vi "Insert Initial Delay - IQ.vi"(0 "data in":T1[](array[typedef])=[{"I"=0.0, "Q"=0.0, "overflow"=FALSE}, {"I"=0.0, "Q"=0.0, "overflow"=FALSE}, {"I"=0.0, "Q"=0.0, "overflow"=FALSE}, {"I"=0.0, "Q"=0.0, "overflow"=FALSE}], 1 "insert":bool, 2 "reset":bool, 9 "input valid":bool, 11 "delay":u32) -> (3 "done":bool, 4 "data out":T1[](array[typedef]), 10 "output valid":bool)   [LabVIEW 2018, in "GettingStarted_5774_FPGA.lvlib"]
doc: "Inserts initial idle samples in the sample stream.\n\nA true on the <B>reset</B> input resets the internal state machine and sets the <B>output valid</B> and <B>done</B> outputs to false. Following a reset the VI waits until it detects a rising edge on the <B>insert</B> input which initiates the idle sample insertion. During this period <B>delay</B> number of idle samples are returned on the <B>data output</B>. When no more idle samples can be returned (because the remaining number of idle samples is less than the number of samples returned on the <B>data out</B> output) the <B>done</B> output is set to true and the VI starts returning the samples provided on the <B>data in</B> input. The <B>data in</B> input is ignored if the <B>done</B> output was false in the previous cycle.\n\nSupported array size of the <B>data in</B> input: 1, 2, 4, 8, 16 or 32.\nThe data pipeline delay of this VI is 1 clock cycle."
uses:
  <instrlib>/_niInstr/DSP/v1/Shared/Public/IQ Data.ctl
  <instrlib>/_niInstr/Basic Elements/v1/FPGA/Private/Count Down U32.vi
  GettingStarted_5774_FPGA.lvlib
  <instrlib>/_niInstr/DSP/v1/Shared/niInstr DSP v1 Shared.lvlib
  <instrlib>/_niInstr/Basic Elements/v1/FPGA/niInstr Basic Elements v1 FPGA.lvlib
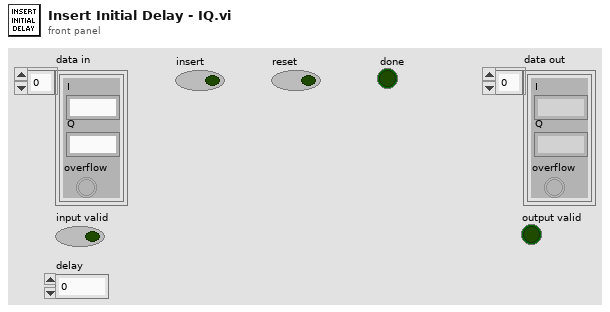
[diagram p1: front panel]
types:
  T1 = typedef "niInstr DSP v1 Shared.lvlib/IQ Data.ctl" = cluster{"I":fxp<+/-,18,1>, "Q":fxp<+/-,18,1>, "overflow":bool}
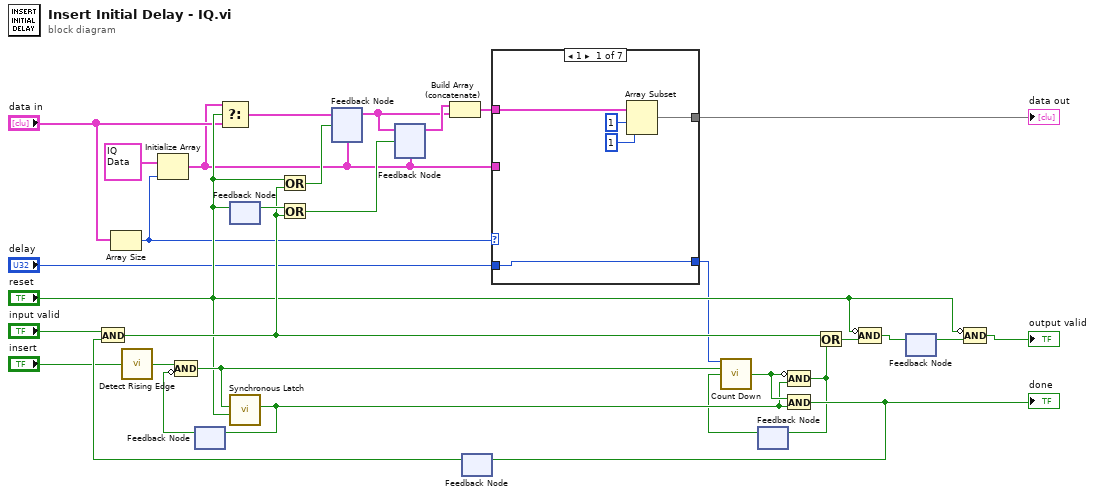
[diagram p0: block diagram]
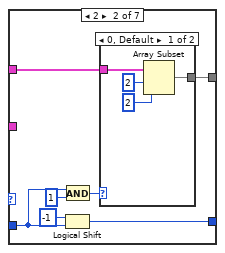
[diagram p2: hidden frame]
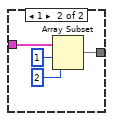
[diagram p3: hidden frame]
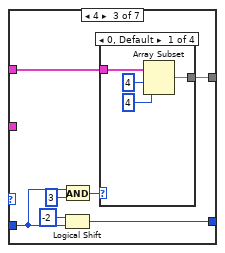
[diagram p4: hidden frame]
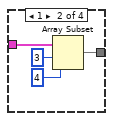
[diagram p5: hidden frame]
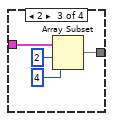
[diagram p6: hidden frame]
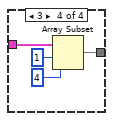
[diagram p7: hidden frame]
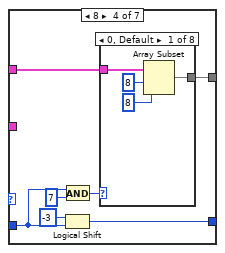
[diagram p8: hidden frame]
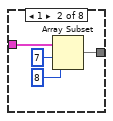
[diagram p9: hidden frame]
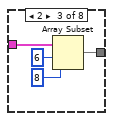
[diagram p10: hidden frame]
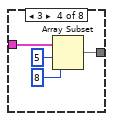
[diagram p11: hidden frame]
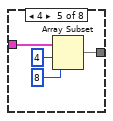
[diagram p12: hidden frame]
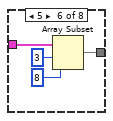
[diagram p13: hidden frame]
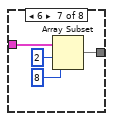
[diagram p14: hidden frame]
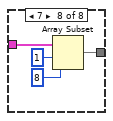
[diagram p15: hidden frame]
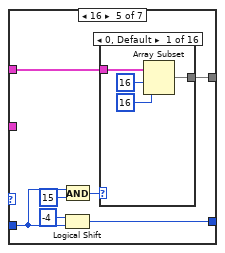
[diagram p16: hidden frame]
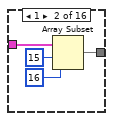
[diagram p17: hidden frame]
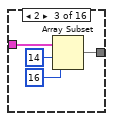
[diagram p18: hidden frame]
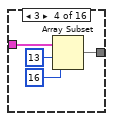
[diagram p19: hidden frame]
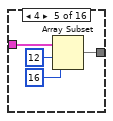
[diagram p20: hidden frame]
diagram:
  n1 = Array Size(array="data in") -> (size(s)=w6:i32)
  n2 = call <instrlib>:"Detect Rising Edge.vi"("signal"="insert") -> ("edge detected"=w19:bool)  [unwired: 14 in]
  n3 = Initialize Array(T1 {"I"=0.0, "Q"=0.0, "overflow"=FALSE} ("data"), w6) -> (w1:T1[])
  n4 = feedback #1() -> (w17:bool)  [unwired: 1 in]
  n5 = Compound Arithmetic op=AND(w19, invert w17) -> (w18:bool)
  n6 = Select(t=w1, s="reset", f="data in") -> (s? t:f=w30:T1[])
  n7 = feedback-in #2("reset") -> ()
  n8 = feedback #2() -> (w27:bool)  [unwired: 1 in]
  n9 = call <instrlib>:"Synchronous Latch.vi"("clear"="reset", "set"=w18) -> ("out"=w16:bool)  [unwired: 9 in]
  n10 = feedback-in #1(w16) -> ()
  n11 = feedback #3(w1) -> (w23:T1[])
  n12 = feedback #4(w1) -> (w24:T1[])
  n13 = Build Array (concatenate)(w24, w23) -> (w4:T1[])
  n14 = feedback #5() -> (w25:bool)  [unwired: 1 in]
  n15 = And(x="input valid", y=w25) -> (x .and. y?=w15:bool)
  n16 = Or(x="reset", y=w15) -> (x .or. y?=w28:bool)
  n17 = Or(x=w27, y=w15) -> (x .or. y?=w26:bool)
  n18 = feedback-in #3(w30, w28) -> ()
  n19 = feedback-in #4(w23, w26) -> ()
  n20 = case shown="1" w6 {
    tunnel: "delay" -> [w34 w42 w57 w80 w119 w190 w324]
    tunnel: w4 -> [w36 w39 w54 w77 w116 w187 _]
    tunnel: [w34 w38 w53 w76 w115 w186 w324] -> w3
    tunnel: [w35 w37 w52 w75 w114 w185 w323] -> w2
    tunnel: w1 -> [_ _ _ _ _ _ w323]
    frame 1 {
      n21 = Array Subset(array=w36, index=1, length=1) -> (w35:T1[])
    }
    frame 2 {
      n22 = Logical Shift(y=i16 -1, x=w42) -> (x << y=w38:u32)
      n23 = And(x=w42, y=u32 1) -> (x .and. y?=w40:u32)
      n24 = case shown="0, Default" w40 {
        tunnel: w39 -> [w47 w51]
        tunnel: [w46 w50] -> w37
        frame 0, Default {
          n25 = Array Subset(array=w47, index=2, length=2) -> (w46:T1[])
        }
        frame 1 {
          n26 = Array Subset(array=w51, index=1, length=2) -> (w50:T1[])
        }
      }
    }
    frame 4 {
      n27 = Logical Shift(y=i16 -2, x=w57) -> (x << y=w53:u32)
      n28 = And(x=w57, y=u32 3) -> (x .and. y?=w55:u32)
      n29 = case shown="0, Default" w55 {
        tunnel: w54 -> [w62 w66 w70 w74]
        tunnel: [w61 w65 w69 w73] -> w52
        frame 0, Default {
          n30 = Array Subset(array=w62, index=4, length=4) -> (w61:T1[])
        }
        frame 1 {
          n31 = Array Subset(array=w66, index=3, length=4) -> (w65:T1[])
        }
        frame 2 {
          n32 = Array Subset(array=w70, index=2, length=4) -> (w69:T1[])
        }
        frame 3 {
          n33 = Array Subset(array=w74, index=1, length=4) -> (w73:T1[])
        }
      }
    }
    frame 8 {
      n34 = Logical Shift(y=i16 -3, x=w80) -> (x << y=w76:u32)
      n35 = And(x=w80, y=u32 7) -> (x .and. y?=w78:u32)
      n36 = case shown="0, Default" w78 {
        tunnel: w77 -> [w85 w89 w93 w97 w101 w105 w109 w113]
        tunnel: [w84 w88 w92 w96 w100 w104 w108 w112] -> w75
        frame 0, Default {
          n37 = Array Subset(array=w85, index=8, length=8) -> (w84:T1[])
        }
        frame 1 {
          n38 = Array Subset(array=w89, index=7, length=8) -> (w88:T1[])
        }
        frame 2 {
          n39 = Array Subset(array=w93, index=6, length=8) -> (w92:T1[])
        }
        frame 3 {
          n40 = Array Subset(array=w97, index=5, length=8) -> (w96:T1[])
        }
        frame 4 {
          n41 = Array Subset(array=w101, index=4, length=8) -> (w100:T1[])
        }
        frame 5 {
          n42 = Array Subset(array=w105, index=3, length=8) -> (w104:T1[])
        }
        frame 6 {
          n43 = Array Subset(array=w109, index=2, length=8) -> (w108:T1[])
        }
        frame 7 {
          n44 = Array Subset(array=w113, index=1, length=8) -> (w112:T1[])
        }
      }
    }
    frame 16 {
      n45 = Logical Shift(y=i16 -4, x=w119) -> (x << y=w115:u32)
      n46 = And(x=w119, y=u32 15) -> (x .and. y?=w117:u32)
      n47 = case shown="0, Default" w117 {
        tunnel: w116 -> [w124 w128 w132 w136 w140 w144 w148 w152 w156 w160 w164 w168 w172 w176 w180 w184]
        tunnel: [w123 w127 w131 w135 w139 w143 w147 w151 w155 w159 w163 w167 w171 w175 w179 w183] -> w114
        frame 0, Default {
          n48 = Array Subset(array=w124, index=16, length=16) -> (w123:T1[])
        }
        frame 1 {
          n49 = Array Subset(array=w128, index=15, length=16) -> (w127:T1[])
        }
        frame 2 {
          n50 = Array Subset(array=w132, index=14, length=16) -> (w131:T1[])
        }
        frame 3 {
          n51 = Array Subset(array=w136, index=13, length=16) -> (w135:T1[])
        }
        frame 4 {
          n52 = Array Subset(array=w140, index=12, length=16) -> (w139:T1[])
        }
        frame 5 {
          n53 = Array Subset(array=w144, index=11, length=16) -> (w143:T1[])
        }
        frame 6 {
          n54 = Array Subset(array=w148, index=10, length=16) -> (w147:T1[])
        }
        frame 7 {
          n55 = Array Subset(array=w152, index=9, length=16) -> (w151:T1[])
        }
        frame 8 {
          n56 = Array Subset(array=w156, index=8, length=16) -> (w155:T1[])
        }
        frame 9 {
          n57 = Array Subset(array=w160, index=7, length=16) -> (w159:T1[])
        }
        frame 10 {
          n58 = Array Subset(array=w164, index=6, length=16) -> (w163:T1[])
        }
        frame 11 {
          n59 = Array Subset(array=w168, index=5, length=16) -> (w167:T1[])
        }
        frame 12 {
          n60 = Array Subset(array=w172, index=4, length=16) -> (w171:T1[])
        }
        frame 13 {
          n61 = Array Subset(array=w176, index=3, length=16) -> (w175:T1[])
        }
        frame 14 {
          n62 = Array Subset(array=w180, index=2, length=16) -> (w179:T1[])
        }
        frame 15 {
          n63 = Array Subset(array=w184, index=1, length=16) -> (w183:T1[])
        }
      }
    }
    frame 32 {
      n64 = Logical Shift(y=i16 -5, x=w190) -> (x << y=w186:u32)
      n65 = And(x=w190, y=u32 31) -> (x .and. y?=w188:u32)
      n66 = case shown="0, Default" w188 {
        tunnel: w187 -> [w195 w199 w203 w207 w211 w215 w219 w223 w227 w231 w235 w239 w243 w247 w251 w255 w259 w263 w267 w271 w275 w279 w283 w287 w291 w295 w299 w303 w307 w311 w315 w319]
        tunnel: [w194 w198 w202 w206 w210 w214 w218 w222 w226 w230 w234 w238 w242 w246 w250 w254 w258 w262 w266 w270 w274 w278 w282 w286 w290 w294 w298 w302 w306 w310 w314 w318] -> w185
        frame 0, Default {
          n67 = Array Subset(array=w195, index=32, length=32) -> (w194:T1[])
        }
        frame 1 {
          n68 = Array Subset(array=w199, index=31, length=32) -> (w198:T1[])
        }
        frame 2 {
          n69 = Array Subset(array=w203, index=30, length=32) -> (w202:T1[])
        }
        frame 3 {
          n70 = Array Subset(array=w207, index=29, length=32) -> (w206:T1[])
        }
        frame 4 {
          n71 = Array Subset(array=w211, index=28, length=32) -> (w210:T1[])
        }
        frame 5 {
          n72 = Array Subset(array=w215, index=27, length=32) -> (w214:T1[])
        }
        frame 6 {
          n73 = Array Subset(array=w219, index=26, length=32) -> (w218:T1[])
        }
        frame 7 {
          n74 = Array Subset(array=w223, index=25, length=32) -> (w222:T1[])
        }
        frame 8 {
          n75 = Array Subset(array=w227, index=24, length=32) -> (w226:T1[])
        }
        frame 9 {
          n76 = Array Subset(array=w231, index=23, length=32) -> (w230:T1[])
        }
        frame 10 {
          n77 = Array Subset(array=w235, index=22, length=32) -> (w234:T1[])
        }
        frame 11 {
          n78 = Array Subset(array=w239, index=21, length=32) -> (w238:T1[])
        }
        frame 12 {
          n79 = Array Subset(array=w243, index=20, length=32) -> (w242:T1[])
        }
        frame 13 {
          n80 = Array Subset(array=w247, index=19, length=32) -> (w246:T1[])
        }
        frame 14 {
          n81 = Array Subset(array=w251, index=18, length=32) -> (w250:T1[])
        }
        frame 15 {
          n82 = Array Subset(array=w255, index=17, length=32) -> (w254:T1[])
        }
        frame 16 {
          n83 = Array Subset(array=w259, index=16, length=32) -> (w258:T1[])
        }
        frame 17 {
          n84 = Array Subset(array=w263, index=15, length=32) -> (w262:T1[])
        }
        frame 18 {
          n85 = Array Subset(array=w267, index=14, length=32) -> (w266:T1[])
        }
        frame 19 {
          n86 = Array Subset(array=w271, index=13, length=32) -> (w270:T1[])
        }
        frame 20 {
          n87 = Array Subset(array=w275, index=12, length=32) -> (w274:T1[])
        }
        frame 21 {
          n88 = Array Subset(array=w279, index=11, length=32) -> (w278:T1[])
        }
        frame 22 {
          n89 = Array Subset(array=w283, index=10, length=32) -> (w282:T1[])
        }
        frame 23 {
          n90 = Array Subset(array=w287, index=9, length=32) -> (w286:T1[])
        }
        frame 24 {
          n91 = Array Subset(array=w291, index=8, length=32) -> (w290:T1[])
        }
        frame 25 {
          n92 = Array Subset(array=w295, index=7, length=32) -> (w294:T1[])
        }
        frame 26 {
          n93 = Array Subset(array=w299, index=6, length=32) -> (w298:T1[])
        }
        frame 27 {
          n94 = Array Subset(array=w303, index=5, length=32) -> (w302:T1[])
        }
        frame 28 {
          n95 = Array Subset(array=w307, index=4, length=32) -> (w306:T1[])
        }
        frame 29 {
          n96 = Array Subset(array=w311, index=3, length=32) -> (w310:T1[])
        }
        frame 30 {
          n97 = Array Subset(array=w315, index=2, length=32) -> (w314:T1[])
        }
        frame 31 {
          n98 = Array Subset(array=w319, index=1, length=32) -> (w318:T1[])
        }
      }
    }
    frame Default {
      n99 = call <instrlib>:"Assert.vi"("assert"=TRUE, "error code"=-1074101118, "enable show error"=TRUE) -> ()  [unwired: 13 in]
    }
  }
  "data out" <- w2
  n100 = feedback #6() -> (w13:bool)  [unwired: 1 in]
  n101 = call-poly <instrlib>:"Count Down.vi"("count in"=w3, "load"=w18, "decrement"=w13) -> ("terminal count"=w21:bool)  [unwired: 11 in, 1 out]
  n102 = And(x=w21, y=w16) -> (x .and. y?=w20:bool)
  "done" <- w20
  n103 = feedback-in #5(w20) -> ()
  n104 = Compound Arithmetic op=AND(invert w21, w16) -> (w12:bool)
  n105 = feedback-in #6(w12) -> ()
  n106 = Or(x=w15, y=w12) -> (x .or. y?=w14:bool)
  n107 = Compound Arithmetic op=AND(invert "reset", w14) -> (w11:bool)
  n108 = feedback-in #7(w11) -> ()
  n109 = feedback #7() -> (w10:bool)  [unwired: 1 in]
  n110 = Compound Arithmetic op=AND(invert "reset", w10) -> (→"output valid":bool)
